vi "Cluster of Limits_UI.vi"(7 "ControlsIndicators":T1, 8 "error in (no error)":errorcluster, 10 "Cluster of limits":refnum<vi>, 11 "Input ListBox Cluster":T7) -> (0 "error out":errorcluster, 3 "ListBox Cluster out":T7)   [LabVIEW 2019, in "ZenGage v3.0 UI.lvclass"]
doc: "This VI checks whether entered Lower Limit, Lower Control Limit values are less than Result value and Upper Limit, Upper Control Limit values are greater then Result value."
uses:
  ZenGage v3.0 UI.lvclass
  Type Definitions/Edit tolerance settings/Edit Tolerance Input.ctl
  Type Definitions/Edit tolerance settings/Rack Selection.ctl
  <vilib>/Utility/miscctls.llb/LVPoint32TypeDef.ctl
  Type Definitions/Controls and Indicators/Select a part (combobox).ctl
  Type Definitions/Controls and Indicators/EDL control references.ctl
  Type Definitions/Controls and Indicators/Diagnostics control referencs.ctl
  Type Definitions/Controls and Indicators/Inspection control references.ctl
  Type Definitions/Controls and Indicators/General_Control references.ctl
  Type Definitions/General/Master sample references.ctl
  Type Definitions/Controls and Indicators/Controls and Indicators Cluster.ctl
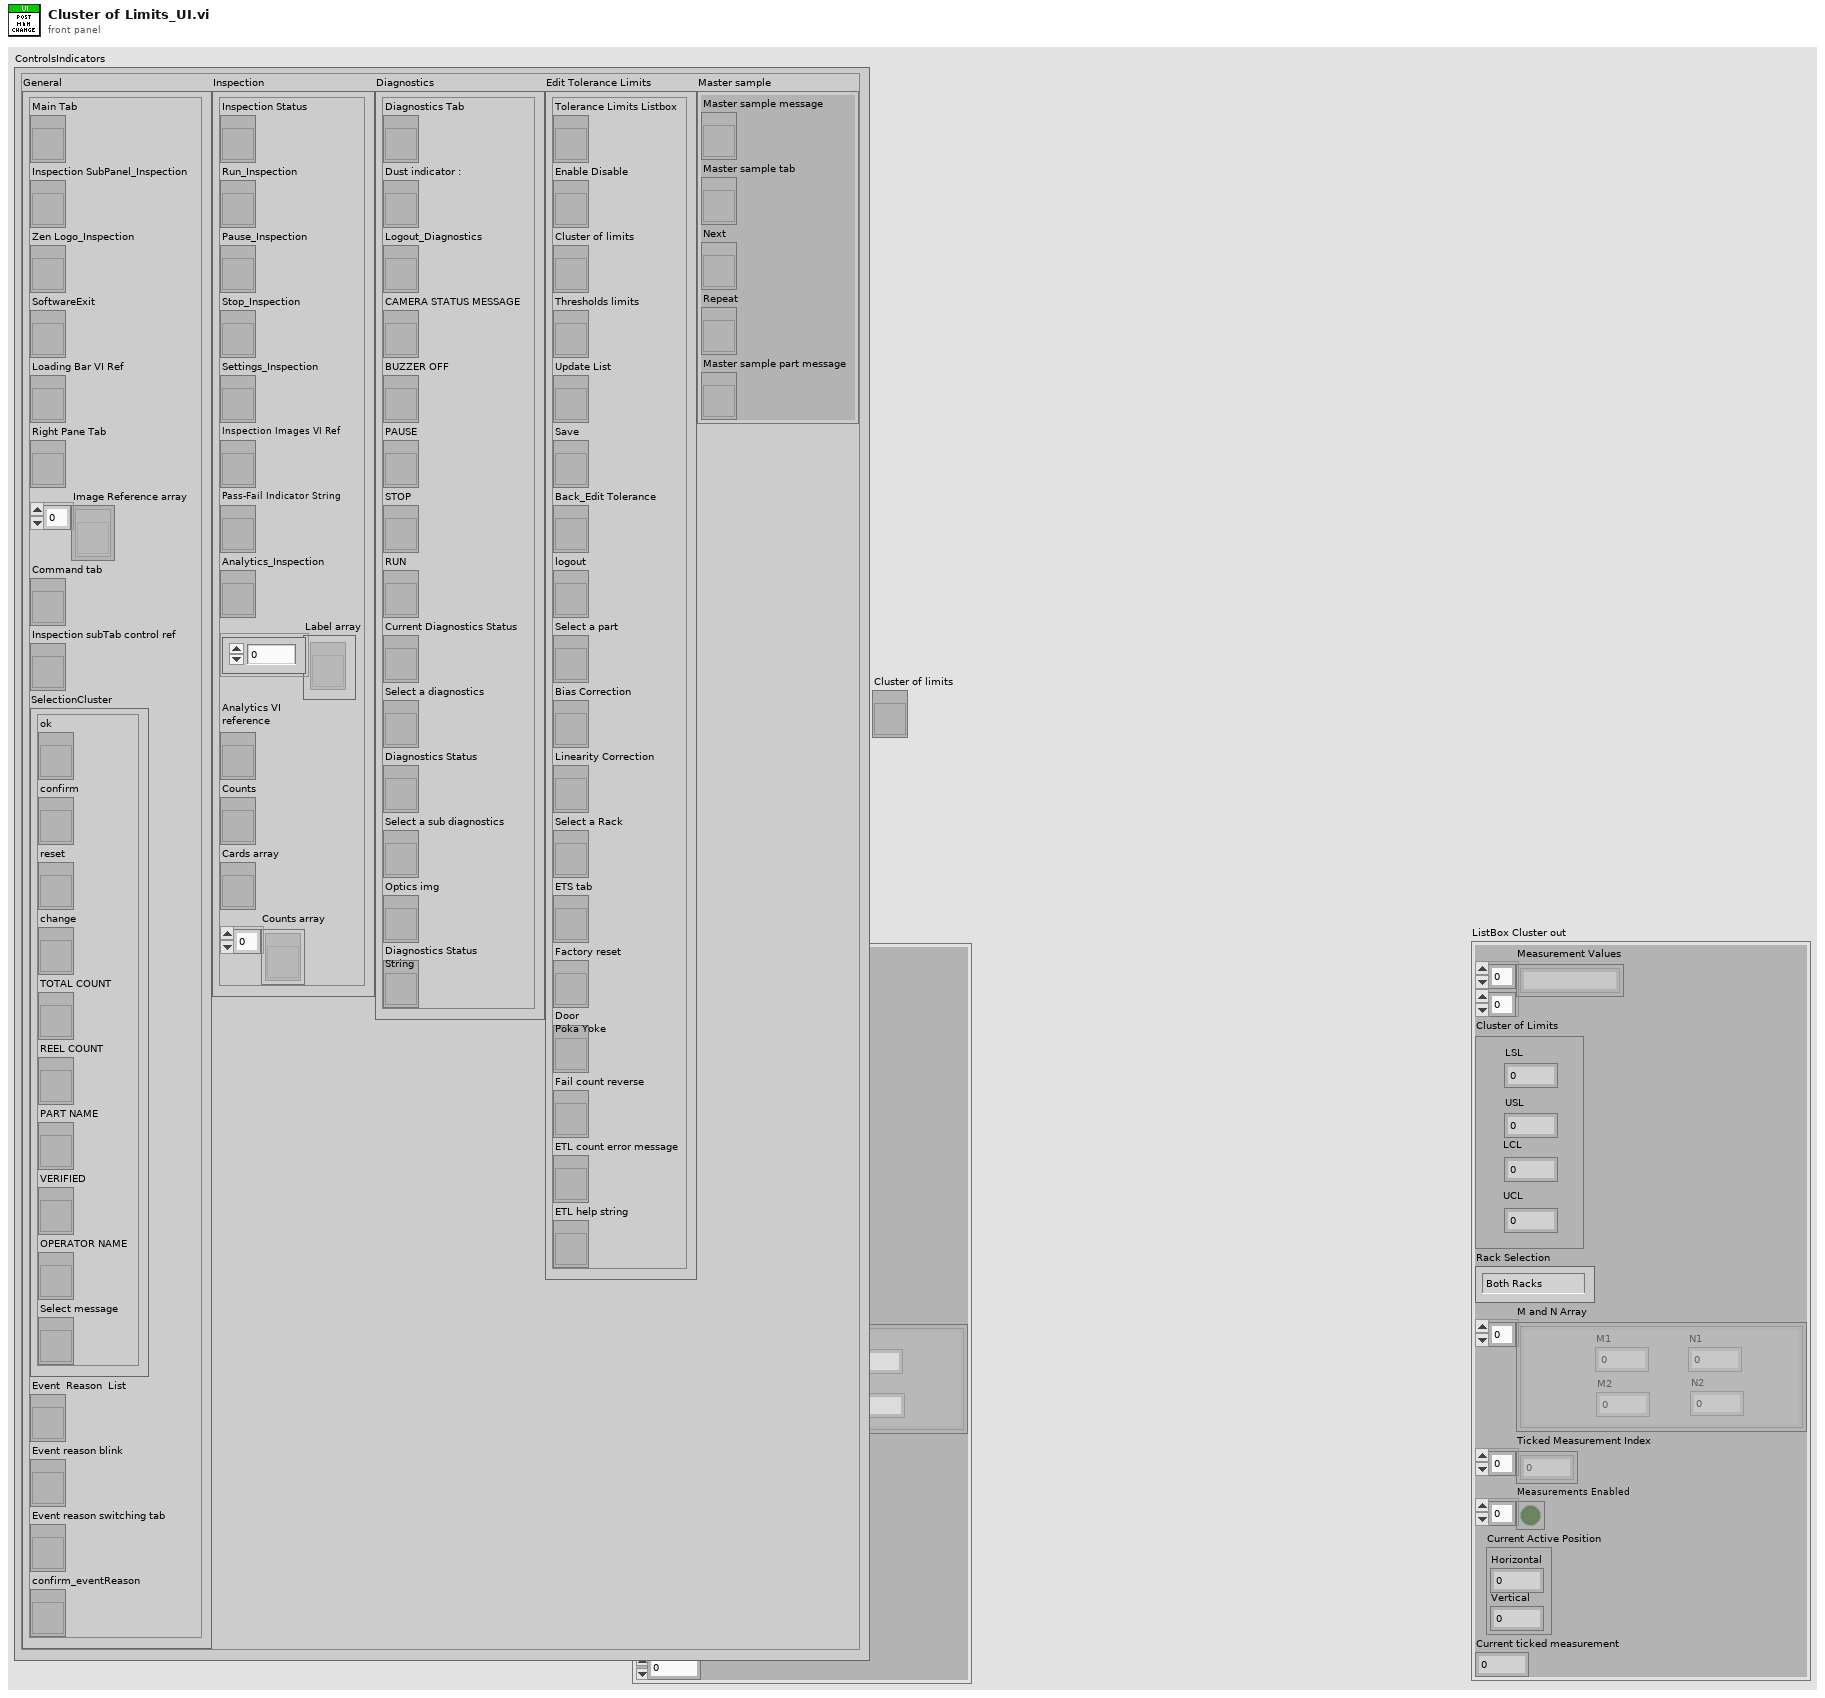
[diagram p1: front panel]
types:
  T1 = typedef "ZenGage v3.0 UI.lvclass/Controls and Indicators Cluster.ctl" = cluster{"General":T2, "Inspection":T3, "Diagnostics":T4, "Edit Tolerance Limits":T5, "Master sample":T6}
  T2 = typedef "ZenGage v3.0 UI.lvclass/General_Control references.ctl" = cluster{"Main Tab":refnum<vi>, "Inspection SubPanel_Inspection":refnum<vi>, "Zen Logo_Inspection":refnum<vi>, "SoftwareExit":refnum<vi>, "Loading Bar VI Ref":refnum<vi>, "Right Pane Tab":refnum<vi>, "Image Reference array":refnum<vi>[], "Command tab":refnum<vi>, "Inspection subTab control ref":refnum<vi>, "SelectionCluster":cluster{"ok":refnum<vi>, "confirm":refnum<vi>, "reset":refnum<vi>, "change":refnum<vi>, "TOTAL COUNT":refnum<vi>, "REEL COUNT":refnum<vi>, "PART NAME":refnum<vi>, "VERIFIED":refnum<vi>, "OPERATOR NAME":refnum<vi>, "Select message":refnum<vi>}, "Event  Reason  List":refnum<vi>, "Event reason blink":refnum<vi>, "Event reason switching tab":refnum<vi>, "confirm_eventReason":refnum<vi>}
  T3 = typedef "ZenGage v3.0 UI.lvclass/Inspection control references.ctl" = cluster{"Inspection Status":refnum<vi>, "Run_Inspection":refnum<vi>, "Pause_Inspection":refnum<vi>, "Stop_Inspection":refnum<vi>, "Settings_Inspection":refnum<vi>, "Inspection Images VI Ref":refnum<vi>, "Pass-Fail Indicator String":refnum<vi>, "Analytics_Inspection":refnum<vi>, "Label array":refnum<vi>[], "Analytics VI\nreference":refnum<vi>, "Counts":refnum<vi>, "Cards array":refnum<vi>, "Counts array":refnum<vi>[]}
  T4 = typedef "ZenGage v3.0 UI.lvclass/Diagnostics control referencs.ctl" = cluster{"Diagnostics Tab":refnum<vi>, "Dust indicator :":refnum<vi>, "Logout_Diagnostics":refnum<vi>, "CAMERA STATUS MESSAGE":refnum<vi>, "BUZZER OFF":refnum<vi>, "PAUSE":refnum<vi>, "STOP":refnum<vi>, "RUN":refnum<vi>, "Current Diagnostics Status":refnum<vi>, "Select a diagnostics":refnum<vi>, "Diagnostics Status":refnum<vi>, "Select a sub diagnostics":refnum<vi>, "Optics img":refnum<vi>, "Diagnostics Status\nString":refnum<vi>}
  T5 = typedef "ZenGage v3.0 UI.lvclass/EDL control references.ctl" = cluster{"Tolerance Limits Listbox":refnum<vi>, "Enable Disable":refnum<vi>, "Cluster of limits":refnum<vi>, "Thresholds limits":refnum<vi>, "Update List":refnum<vi>, "Save":refnum<vi>, "Back_Edit Tolerance":refnum<vi>, "logout":refnum<vi>, "Select a part":refnum<vi>, "Bias Correction":refnum<vi>, "Linearity Correction":refnum<vi>, "Select a Rack":refnum<vi>, "ETS tab":refnum<vi>, "Factory reset":refnum<vi>, "Door\nPoka Yoke":refnum<vi>, "Fail count reverse":refnum<vi>, "ETL count error message":refnum<vi>, "ETL help string":refnum<vi>}
  T6 = typedef "Master sample references.ctl" = cluster{"Master sample message":refnum<vi>, "Master sample tab":refnum<vi>, "Next":refnum<vi>, "Repeat":refnum<vi>, "Master sample part message":refnum<vi>}
  T7 = typedef "ZenGage v3.0 UI.lvclass/Edit Tolerance Input.ctl" = cluster{"Measurement Values":string[][], "Cluster of Limits":cluster{"LSL":dbl, "USL":dbl, "LCL":dbl, "UCL":dbl}, "Rack Selection":T8, "M and N Array":cluster{"M1":u64, "M2":u64, "N1":u64, "N2":u64}[], "Ticked Measurement Index":u32[], "Measurements Enabled":bool[], "Current Active Position":T9, "Current ticked measurement":dbl}
  T8 = typedef "ZenGage v3.0 UI.lvclass/Rack Selection.ctl" = enum16{"Both Racks", "Rack 2", "Rack 1"}
  T9 = typedef "LVPoint32TypeDef.ctl" = cluster{"Horizontal":i32, "Vertical":i32}
  T10 = cluster{"Lower Limit":dbl, "Upper Limit":dbl, "Lower Control Limit":dbl, "Upper Control Limit":dbl}
  T11 = enum8{"Enabled", "Disabled", "Disabled and Grayed Out"}
  T12 = cluster{"LSL":dbl, "USL":dbl, "LCL":dbl, "UCL":dbl}
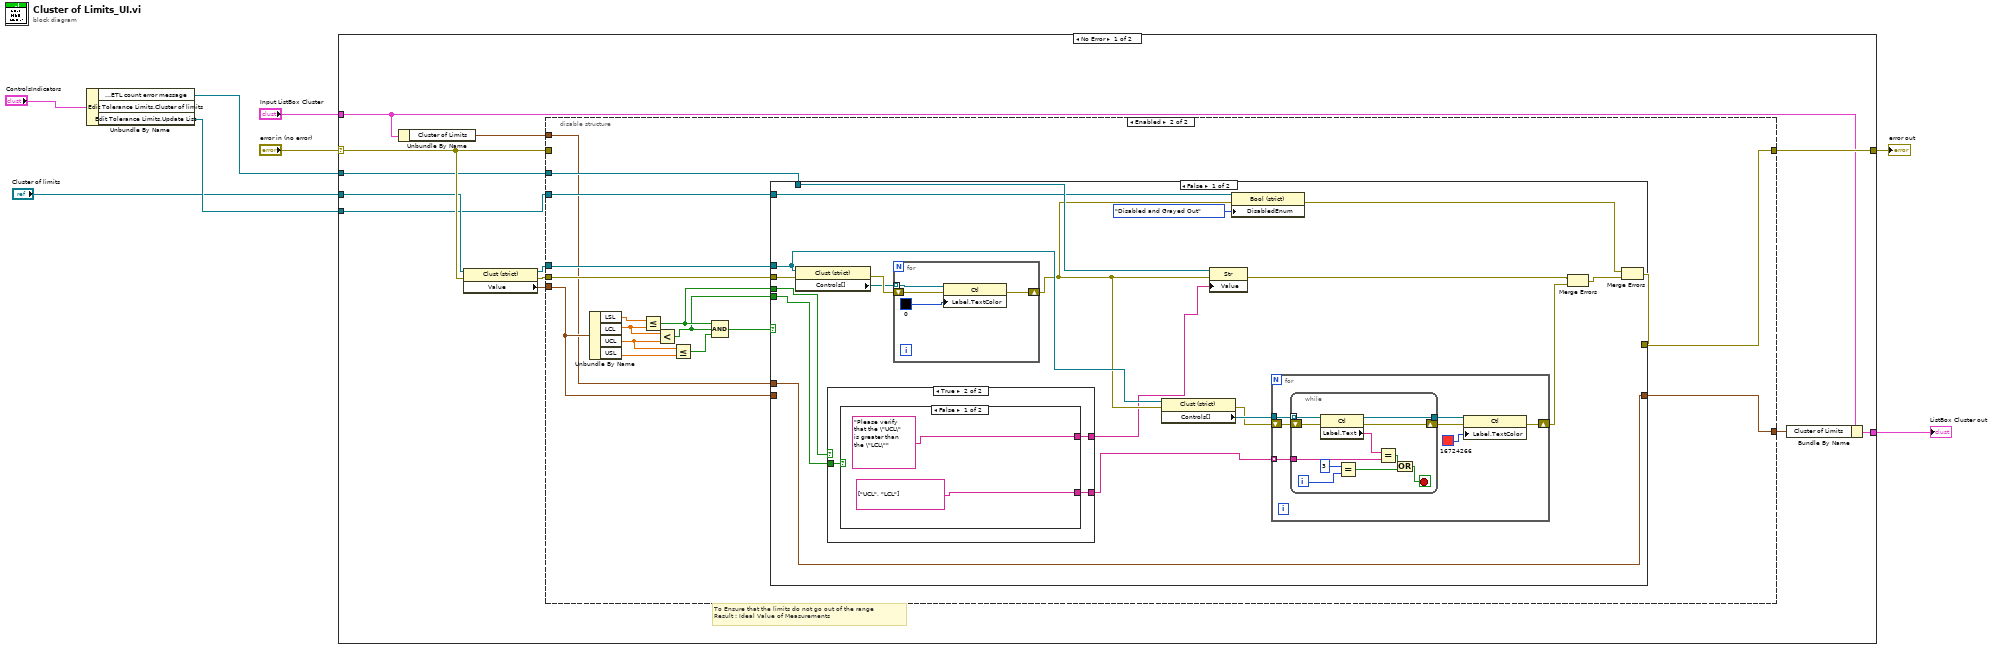
[diagram p0: block diagram]
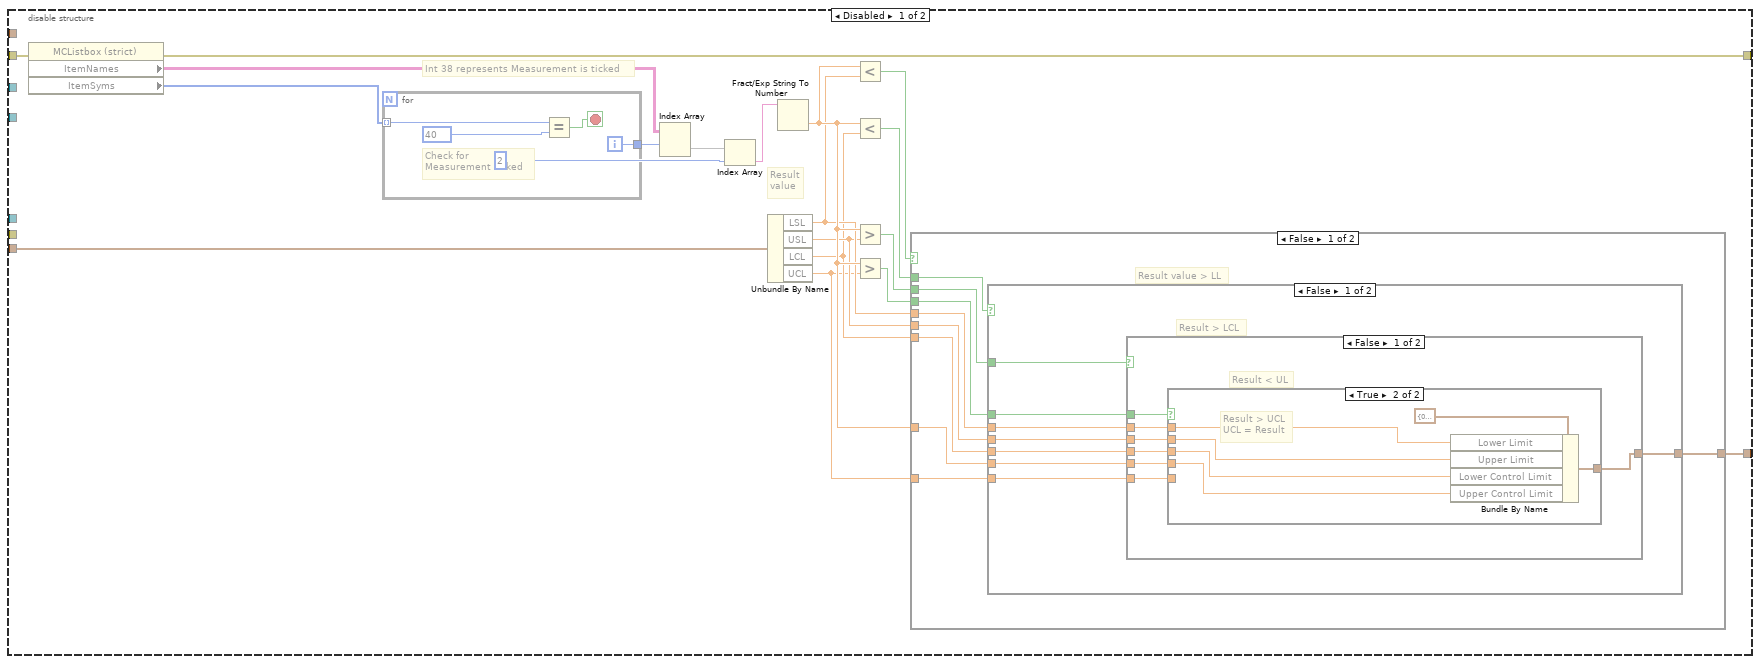
[diagram p2: hidden frame]
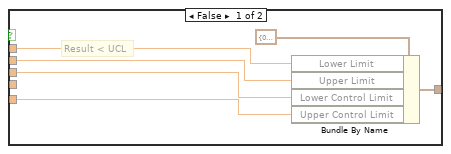
[diagram p3: hidden frame]
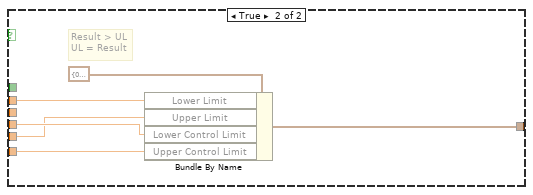
[diagram p4: hidden frame]
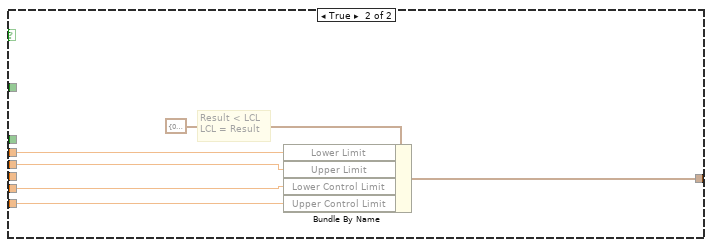
[diagram p5: hidden frame]
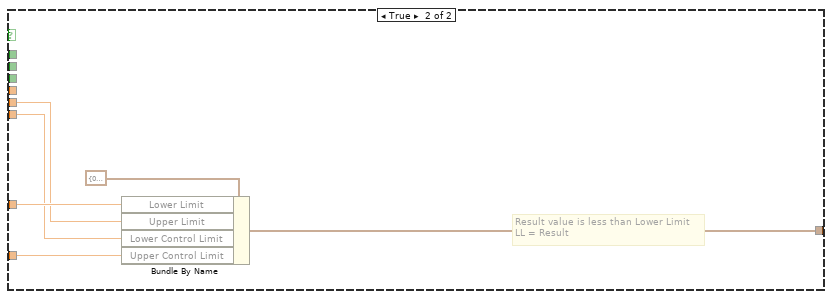
[diagram p6: hidden frame]
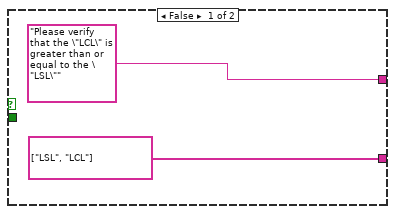
[diagram p7: hidden frame]
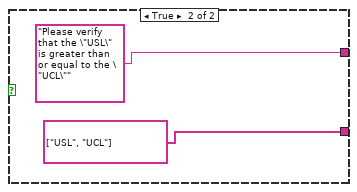
[diagram p8: hidden frame]
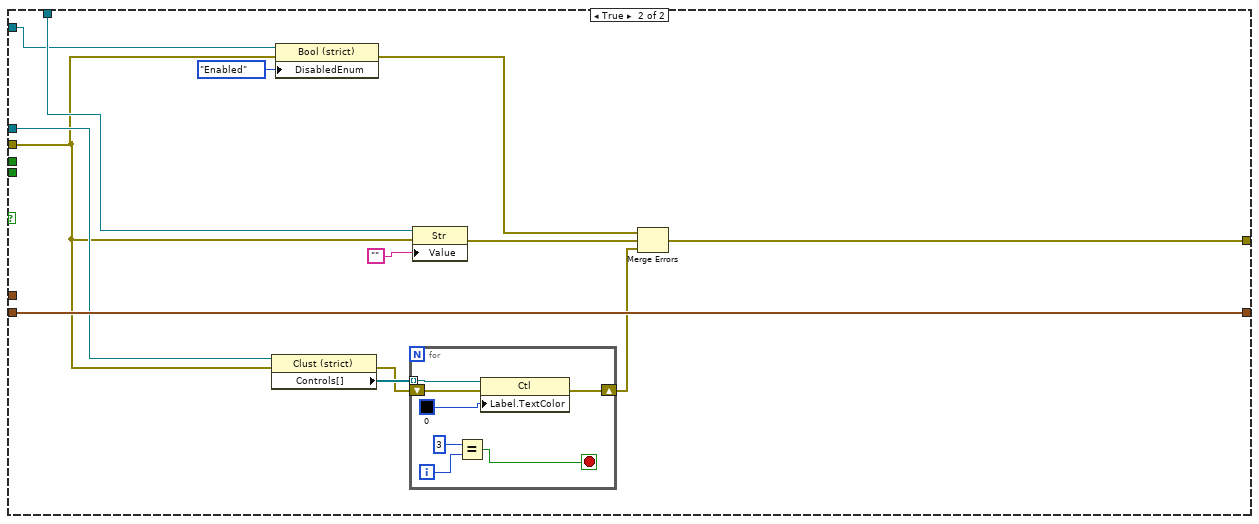
[diagram p9: hidden frame]
diagram:
  n1 = Unbundle By Name("ControlsIndicators") -> ("Edit Tolerance Limits.ETL count error message"=w3:refnum<vi>, "Edit Tolerance Limits.Update List"=w2:refnum<vi>)  [unwired: 1 out]
  n2 = case shown="No Error" "error in (no error)" {
    selector: "error in (no error)" -> [w17 w186]
    tunnel: [w19 w186] -> w7
    tunnel: [w18 w185] -> w5
    tunnel: "Input ListBox Cluster" -> [w13 w185]
    tunnel: "Cluster of limits" -> [w10 _]
    tunnel: w3 -> [w14 _]
    tunnel: w2 -> [w9 _]
    frame No Error {
      # "To Ensure that the limits do not go out of the range\nResult : Ideal Value of Measurements"
      n3 = Unbundle By Name(w13) -> ("Cluster of Limits"=w12:T12)
      n4 = property class="Clust (strict)"(reference=w10, error in=w17) -> (reference out=w11:refnum<vi>, error out=w15:errorcluster, "Value"=w16:T12)
      n5 = disable-structure shown="Enabled" {
        disable-tunnel: [w24 w112] -> w20
        disable-tunnel: [w23 w109] -> w19
        disable-tunnel: w17 -> [w22 _]
        disable-tunnel: w16 -> [w21 w113]
        disable-tunnel: w15 -> [_ w111]
        disable-tunnel: w14 -> [_ w110]
        disable-tunnel: w12 -> [_ w106]
        disable-tunnel: w11 -> [_ w108]
        disable-tunnel: w9 -> [_ w107]
        frame Disabled {
          # "Result\nvalue"
          # "Int 38 represents Measurement is ticked"
          n6 = property class="MCListbox (strict)"(error in=w22) -> (error out=w23:errorcluster, "ItemNames"=w37:string[][], "ItemSyms"=w39:i32[])  [unwired: 1 in, 1 out]
          n7 = for {
            tunnel: w39 -> [w97] mode=indexing
            tunnel: [w95] -> w38
            i -> [w95]
            stop <- w96 stop-if-true
            # "Check for \nMeasurement ticked"
            n8 = Equal?(x=w97, y=40) -> (x = y?=w96:bool)
          }
          n9 = Index Array(array=w37, index (row)=w38) -> (element=w30:string[])  [unwired: 1 in]
          n10 = Index Array(array=w30, index=2) -> (element=w35:string)
          n11 = Unbundle By Name(w21) -> ("LSL"=w28:dbl, "USL"=w27:dbl, "LCL"=w26:dbl, "UCL"=w25:dbl)
          n12 = Fract/Exp String To Number(string=w35) -> (number=w29:dbl)  [unwired: 3 in, 1 out]
          n13 = Less?(x=w29, y=w28) -> (x < y?=w34:bool)
          n14 = Less?(x=w29, y=w26) -> (x < y?=w33:bool)
          n15 = Greater?(x=w29, y=w27) -> (0:w32:bool)
          n16 = Greater?(x=w29, y=w25) -> (0:w31:bool)
          n17 = case shown="False" w34 {
            tunnel: w27 -> [w48 w91]
            tunnel: w25 -> [w47 w89]
            tunnel: w28 -> [w46 _]
            tunnel: w26 -> [w45 w90]
            tunnel: w29 -> [w43 w92]
            tunnel: w33 -> [w44 _]
            tunnel: w32 -> [w42 _]
            tunnel: w31 -> [w41 _]
            tunnel: [w40 w88] -> w24
            frame False {
              # "Result value > LL"
              n18 = case shown="False" w44 {
                tunnel: w48 -> [w56 w83]
                tunnel: w47 -> [w55 w84]
                tunnel: w46 -> [w54 w85]
                tunnel: w45 -> [w53 _]
                tunnel: w43 -> [w51 w86]
                tunnel: w42 -> [w52 _]
                tunnel: w41 -> [w50 _]
                tunnel: [w49 w82] -> w40
                frame False {
                  # "Result > LCL"
                  n19 = case shown="False" w52 {
                    tunnel: w56 -> [w63 _]
                    tunnel: w55 -> [w62 w78]
                    tunnel: w54 -> [w58 w80]
                    tunnel: w53 -> [w61 w79]
                    tunnel: w51 -> [w59 w77]
                    tunnel: w50 -> [w60 _]
                    tunnel: [w57 w76] -> w49
                    frame False {
                      # "Result < UL"
                      n20 = case shown="True" w60 {
                        tunnel: w63 -> [w67 w72]
                        tunnel: w62 -> [w65 _]
                        tunnel: w58 -> [w68 w73]
                        tunnel: w61 -> [w66 w71]
                        tunnel: w59 -> [_ w74]
                        tunnel: [w64 w70] -> w57
                        frame False {
                          # "Result < UCL"
                          n21 = Bundle By Name(cluster=T10 {"Lower Limit"=0.0, "Upper Limit"=0.0, "Lower Control Limit"=0.0, "Upper Control Limit"=0.0} ("Value"), "Lower Limit"=w68, "Upper Limit"=w67, "Lower Control Limit"=w66, "Upper Control Limit"=w65) -> (w64:T10)
                        }
                        frame True {
                          # "Result > UCL\nUCL = Result"
                          n22 = Bundle By Name(cluster=T10 {"Lower Limit"=0.0, "Upper Limit"=0.0, "Lower Control Limit"=0.0, "Upper Control Limit"=0.0} ("Value"), "Lower Limit"=w73, "Upper Limit"=w72, "Lower Control Limit"=w71, "Upper Control Limit"=w74) -> (w70:T10)
                        }
                      }
                    }
                    frame True {
                      # "Result > UL\nUL = Result"
                      n23 = Bundle By Name(cluster=T10 {"Lower Limit"=0.0, "Upper Limit"=0.0, "Lower Control Limit"=0.0, "Upper Control Limit"=0.0} ("Value"), "Lower Limit"=w80, "Upper Limit"=w77, "Lower Control Limit"=w79, "Upper Control Limit"=w78) -> (w76:T10)
                    }
                  }
                }
                frame True {
                  # "Result < LCL\nLCL = Result"
                  n24 = Bundle By Name(cluster=T10 {"Lower Limit"=0.0, "Upper Limit"=0.0, "Lower Control Limit"=0.0, "Upper Control Limit"=0.0} ("Value"), "Lower Limit"=w85, "Upper Limit"=w83, "Lower Control Limit"=w86, "Upper Control Limit"=w84) -> (w82:T10)
                }
              }
            }
            frame True {
              # "Result value is less than Lower Limit\nLL = Result"
              n25 = Bundle By Name(cluster=T10 {"Lower Limit"=0.0, "Upper Limit"=0.0, "Lower Control Limit"=0.0, "Upper Control Limit"=0.0} ("Value"), "Lower Limit"=w92, "Upper Limit"=w91, "Lower Control Limit"=w90, "Upper Control Limit"=w89) -> (w88:T10)
            }
          }
        }
        frame Enabled {
          n26 = Unbundle By Name(w113) -> ("LSL"=w105:dbl, "LCL"=w104:dbl, "UCL"=w103:dbl, "USL"=w102:dbl)
          n27 = Less Or Equal?(x=w105, y=w104) -> (x <= y?=w100:bool)
          n28 = Less?(x=w104, y=w103) -> (x < y?=w99:bool)
          n29 = Less Or Equal?(x=w103, y=w102) -> (x <= y?=w98:bool)
          n30 = Compound Arithmetic op=AND(w100, w99, w98) -> (w101:bool)
          n31 = case shown="False" w101 {
            tunnel: w113 -> [_ w177]
            tunnel: [w132 w177] -> w112
            tunnel: w111 -> [w124 w166]
            tunnel: w110 -> [w133 w173]
            tunnel: w106 -> [w132 _]
            tunnel: [w129 w169] -> w109
            tunnel: w108 -> [w123 w174]
            tunnel: w107 -> [w131 w167]
            tunnel: w100 -> [w117 _]
            tunnel: w99 -> [w114 _]
            frame False {
              n32 = property class="Clust (strict)"(reference=w123, error in=w124) -> (error out=w126:errorcluster, "Controls[]"=w125:refnum<vi>[])  [unwired: 1 out]
              n33 = case shown="True" w117 {
                tunnel: [string[] ["LSL", "LCL"] w137] -> w115
                tunnel: ["Please verify that the \"LCL\" is greater than or equal to the \"LSL\"" w136] -> w116
                tunnel: w114 -> [_ w138]
                frame False {
                }
                frame True {
                  n34 = case shown="False" w138 {
                    tunnel: [string[] ["UCL", "LCL"] string[] ["USL", "UCL"]] -> w137
                    tunnel: ["Please verify that the \"UCL\" is greater than the \"LCL\"" "Please verify that the \"USL\" is greater than or equal to the \"UCL\""] -> w136
                    frame False {
                    }
                    frame True {
                    }
                  }
                }
              }
              n35 = for {
                tunnel: w125 -> [w162] mode=indexing
                shift-right: [w161] -> w122
                shift-left: w126 -> [w163]
                n36 = property class="Ctl"(reference=w162, error in=w163, "Label.TextColor"=u32 0) -> (error out=w161:errorcluster)  [unwired: 1 out]
              }
              n37 = property class="Clust (strict)"(reference=w123, error in=w122) -> (error out=w120:errorcluster, "Controls[]"=w121:refnum<vi>[])  [unwired: 1 out]
              n38 = property class="Str"(reference=w133, error in=w122, "Value"=w116) -> (error out=w119:errorcluster)  [unwired: 1 out]
              n39 = property class="Bool (strict)"(reference=w131, error in=w122, "DisabledEnum"=T11."Disabled and Grayed Out" ("Disabled")) -> (error out=w128:errorcluster)  [unwired: 1 out]
              n40 = for {
                tunnel: w121 -> [w149]
                shift-right: [w145] -> w118
                shift-left: w120 -> [w148]
                tunnel: w115 -> [w147] mode=indexing
                n41 = while {
                  tunnel: w149 -> [w160] mode=indexing
                  shift-right: [w158] -> w146
                  shift-left: w148 -> [w159]
                  tunnel: w147 -> [w156]
                  tunnel: [w155] -> w144
                  i -> [w151]
                  stop <- w150 stop-if-true
                  n42 = property class="Ctl"(reference=w160, error in=w159) -> (reference out=w155:refnum<vi>, error out=w158:errorcluster, "Label.Text"=w157:string)
                  n43 = Equal?(x=3, y=w151) -> (x = y?=w154:bool)
                  n44 = Equal?(x=w157, y=w156) -> (x = y?=w152:bool)
                  n45 = Or(x=w152, y=w154) -> (x .or. y?=w150:bool)
                }
                n46 = property class="Ctl"(reference=w144, error in=w146, "Label.TextColor"=u32 16724266) -> (error out=w145:errorcluster)  [unwired: 1 out]
              }
              n47 = Merge Errors(w119, w118) -> (w130:errorcluster)
              n48 = Merge Errors(w128, w130) -> (w129:errorcluster)
            }
            frame True {
              n49 = property class="Clust (strict)"(reference=w174, error in=w166) -> (error out=w175:errorcluster, "Controls[]"=w176:refnum<vi>[])  [unwired: 1 out]
              n50 = property class="Bool (strict)"(reference=w167, error in=w166, "DisabledEnum"=T11."Enabled" ("Disabled")) -> (error out=w165:errorcluster)  [unwired: 1 out]
              n51 = for {
                tunnel: w176 -> [w182] mode=indexing
                shift-right: [w181] -> w170
                shift-left: w175 -> [w183]
                i -> [w179]
                stop <- w178 stop-if-true
                n52 = Equal?(x=3, y=w179) -> (x = y?=w178:bool)
                n53 = property class="Ctl"(reference=w182, error in=w183, "Label.TextColor"=u32 0) -> (error out=w181:errorcluster)  [unwired: 1 out]
              }
              n54 = property class="Str"(reference=w173, error in=w166, "Value"="") -> (error out=w171:errorcluster)  [unwired: 1 out]
              n55 = Merge Errors(w165, w171, w170) -> (w169:errorcluster)
            }
          }
        }
      }
      n56 = Bundle By Name(cluster=w13, "Cluster of Limits"=w20) -> (w18:T7)
    }
    frame Error {
    }
  }
  "error out" <- w7
  "ListBox Cluster out" <- w5
